vi "sort 1D array with index (SubVI).vi"(11 "input":dbl[](array[numeric])) -> (2 "indices":i32[](array[numeric]), 3 "sorted array":dbl[](array[numeric]))   [LabVIEW 2024]
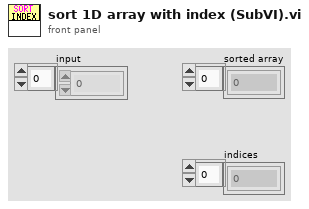
[diagram p1: front panel]
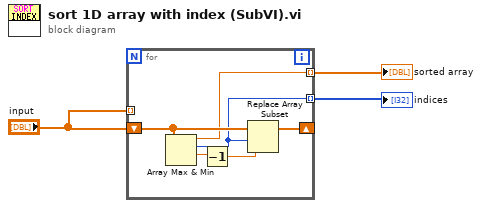
[diagram p0: block diagram]
diagram:
  n1 = for {
    tunnel: "input" -> [_] mode=indexing
    shift-right: [w9] -> _
    shift-left: "input" -> [w8]
    tunnel: [w5] -> w3 mode=indexing
    tunnel: [w4] -> w2 mode=indexing
    n2 = Array Max & Min(array=w8) -> (max value=w4:dbl, max index (indices)=w5:i32, min value=w6:dbl)  [unwired: 1 out]
    n3 = Decrement(x=w6) -> (x-1=w7:dbl)
    n4 = Replace Array Subset(array=w8, new element=w7, index=w5) -> (w9:dbl[])
  }
  "indices" <- w3
  "sorted array" <- w2
